vi "PhidgetEnableServerDiscovery.vi"(8 "error in":errorcluster) -> (0 "error out":errorcluster)   [LabVIEW 2012, in "Phidget Common.lvlib"]
doc: "${EnableServerDiscovery:Header}"
uses:
  <instrlib>/Phidgets/Phidget Common/Phidget Common.lvlib
  phidget22.dll
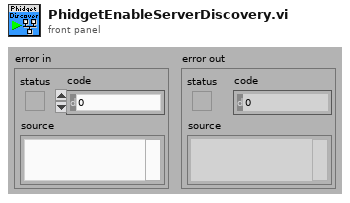
[diagram p1: front panel]
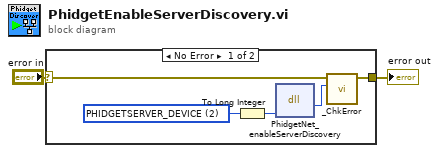
[diagram p0: block diagram]
diagram:
  n1 = case shown="No Error" "error in" {
    selector: "error in" -> [w7 w8]
    tunnel: [w5 w8] -> w1
    frame No Error {
      w3 = u32 2 items=["PHIDGETSERVER_NONE", "PHIDGETSERVER_DEVICELISTENER", "PHIDGETSERVER_DEVICE", "PHIDGETSERVER_DEVICEREMOTE", "PHIDGETSERVER_DICTIONARYLISTENER", "PHIDGETSERVER_DICTIONARY", "PHIDGETSERVER_DICTIONARYREMOTE", "PHIDGETSERVER_WWWLISTENER", "PHIDGETSERVER_WWW", "PHIDGETSERVER_WWWREMOTE", "PHIDGETSERVER_SBC"] ("srvt")
      n2 = To Long Integer(number=w3) -> (32bit integer=w4:i32)
      n3 = dll-call lib="phidget22.dll" fn="PhidgetNet_enableServerDiscovery"("srvt"=w4) -> ("return type"=w6:i32)  [unwired: 4 in, 2 out]
      n4 = call <instrlib>:"_ChkError.vi"("Return Code"=w6, "error in (no error)"=w7) -> ("error out"=w5:errorcluster)  [unwired: 9 in]
    }
    frame Error {
    }
  }
  "error out" <- w1
